vi "get speed.vi"(8 "error in (no error)":errorcluster, 10 "Device Number":i8=1, 11 "VISA resource name":refnum<visa-resource-name>) -> (0 "error out":errorcluster, 2 "Data":i32, 3 "VISA resource name out":refnum<visa-resource-name>)   [LabVIEW 2020]
uses:
  Response.ctl
  ZaberTSeries.lvlib
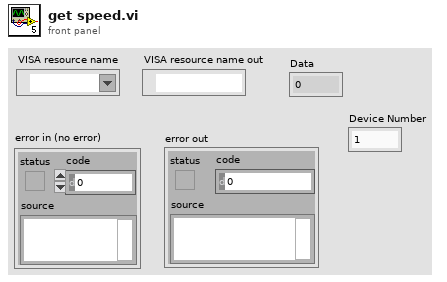
[diagram p1: front panel]
types:
  T1 = typedef "ZaberTSeries.lvlib/Response.ctl" = cluster{"Device Number":u8, "Command":u8, "Data":i32}
  T2 = cluster{"Device Number":i8, "Command":u8, "Data":i32, "Response Count":i32}
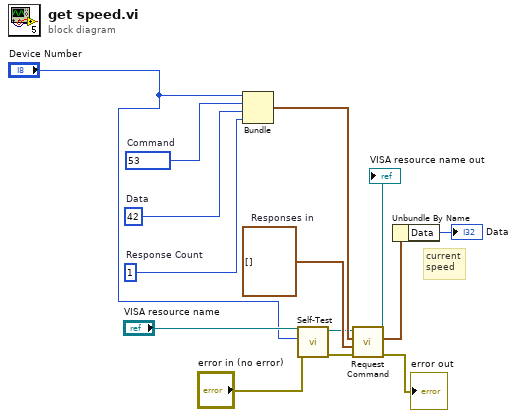
[diagram p0: block diagram]
diagram:
  w11 = 42  # Data
  w12 = 1  # Response Count
  w13 = u8 53 items=["Echo"=55, "Home"=1, "Move Absolute"=20, "Move Relative"=21, "Move at Constant Speed"=22, "Renumber"=2, "Restore Settings"=36, "Stop"=23]  # Command
  w10 = T1[] []  # Responses in
  # "current\nspeed"
  n1 = Bundle("Device Number"="Device Number", "Command"=w13, "Data"=w11, "Response Count"=w12) -> (w8:T2)  [unwired: 1 in]
  n2 = call "Self-Test.vi"("error in (no error)"="error in (no error)", "Device Number"="Device Number", "VISA resource name"="VISA resource name") -> ("error out"=w7:errorcluster, "VISA resource name out"=w6:refnum<visa-resource-name>)  [unwired: 5 in, 2 out]
  n3 = call "Request Command.vi"("error in (no error)"=w7, "Responses in"=w10, "Request"=w8, "VISA resource name"=w6) -> ("error out"=→"error out":errorcluster, "First Response"=w9:T1, "VISA resource name out"=→"VISA resource name out":refnum<visa-resource-name>)  [unwired: 4 in, 1 out]
  n4 = Unbundle By Name(w9) -> ("Data"=→"Data":i32)
